vi "load_validation_file.vi"(6 "LUA Validation File":path, 10 "Parameters Tree":refnum<vi>) -> (2 "Vali File Loaded":bool, 3 "# Lines":i32)   [LabVIEW 2019]
uses:
  lib/libSpecValiReader.so
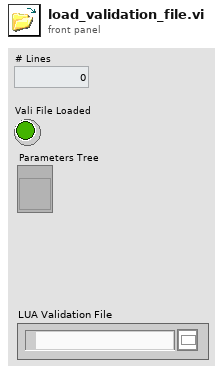
[diagram p1: front panel]
types:
  T1 = cluster{string, string[], "Child Tag":string, i32, "Child Only?":bool, i32}
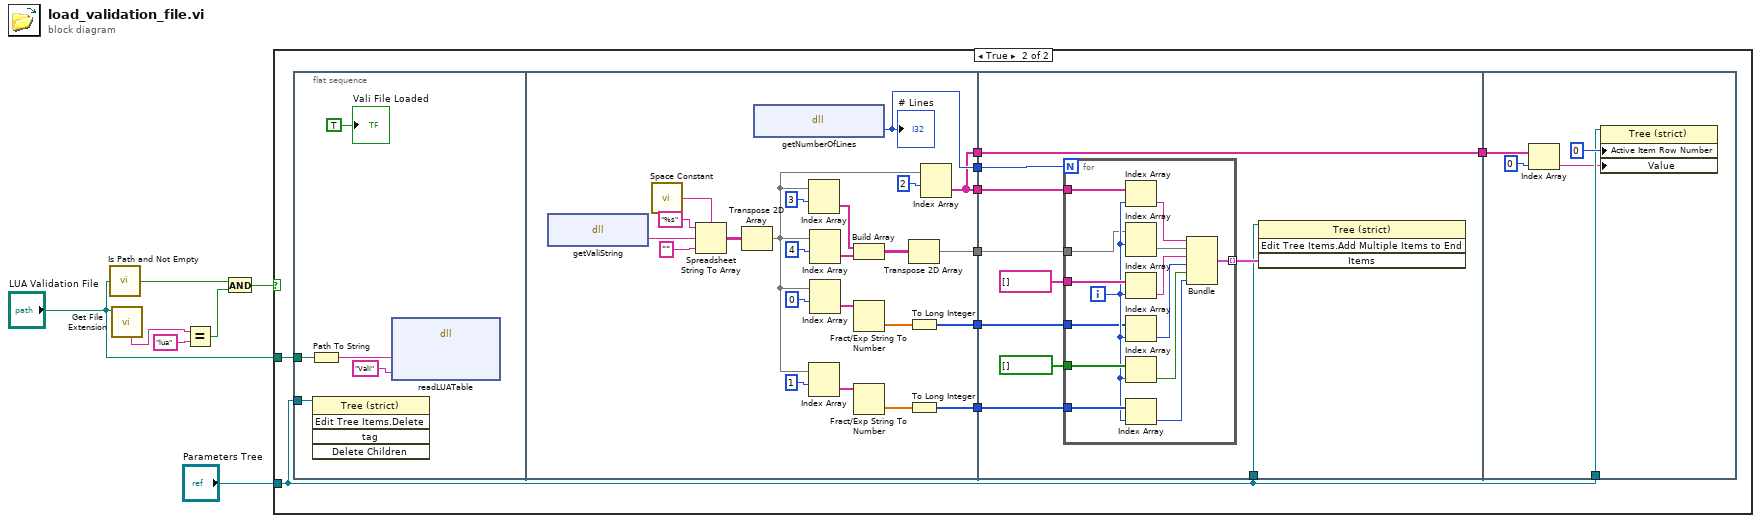
[diagram p0: block diagram]
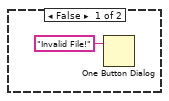
[diagram p2: hidden frame]
diagram:
  n1 = call <vilib>:"Is Path and Not Empty.vi"("path"="LUA Validation File") -> ("Is Path and Not Empty?"=w3:bool)  [unwired: 4 in]
  n2 = call <vilib>:"Get File Extension.vi"("file"="LUA Validation File") -> ("unmodified file extension"=w6:string)  [unwired: 6 in, 4 out]
  n3 = Equal?(x=w6, y="lua") -> (x = y?=w2:bool)
  n4 = And(x=w3, y=w2) -> (x .and. y?=w1:bool)
  n5 = case shown="True" w1 {
    tunnel: "Parameters Tree" -> [_ w10]
    tunnel: "LUA Validation File" -> [_ w9]
    frame False {
      n6 = One Button Dialog(message="Invalid File!") -> ()  [unwired: 1 in, 1 out]
    }
    frame True {
      n7 = flat-sequence {
        tunnel: w10 -> [w20]
        tunnel: w9 -> [w18]
        tunnel: [w41] -> w17
        tunnel: [w36] -> w16
        tunnel: [w32] -> w15
        tunnel: [w25] -> w14
        tunnel: [w25] -> w13
        tunnel: [w23] -> w12
        tunnel: w17 -> [w52]
        tunnel: w10 -> [w51]
        tunnel: w16 -> [w50]
        tunnel: w15 -> [w49]
        tunnel: w14 -> [w48]
        tunnel: [w47] -> w11
        tunnel: w13 -> [w47]
        tunnel: w12 -> [w46]
        tunnel: w10 -> [w72]
        tunnel: w11 -> [w71]
        frame #0 {
          n8 = Path To String(path=w18) -> (string=w19:string)
          n9 = invoke on="Invoke Node" class="Tree (strict)" method="Edit Tree Items.Delete"(reference=w20) -> ()  [unwired: 4 in, 5 out]
          n10 = dll-call lib="home/paul/Schreibtisch/Biogas_plant_setup/lib/libSpecValiReader.so" fn="readLUATable"("filename"=w19, "vali_or_spec"="Vali" ("spec_filename")) -> ()  [unwired: 6 in, 2 out]
          "Vali File Loaded" <- TRUE ("Vali File Loaded")
        }
        frame #1 {
          n11 = dll-call lib="home/paul/Schreibtisch/Biogas_plant_setup/lib/libSpecValiReader.so" fn="getValiString"() -> ("return type"=w45:string)  [unwired: 3 in, 2 out]
          n12 = call <vilib>:"Space Constant.vi"() -> ("String"=w40:string)
          n13 = Spreadsheet String To Array(delimiter (Tab)=w40, format string="%s", spreadsheet string=w45, array type (2D Dbl)="") -> (array=w42:string[][])
          n14 = Transpose 2D Array(2D array=w42) -> (transposed array=w29:string[][])
          n15 = dll-call lib="home/paul/Schreibtisch/Biogas_plant_setup/lib/libSpecValiReader.so" fn="getNumberOfLines"() -> ("numLines"=w41:i32)  [unwired: 3 in, 2 out]
          "# Lines" <- w41
          n16 = Index Array(array=w29, index (row)=3) -> (element=w27:string[])  [unwired: 1 in]
          n17 = Index Array(array=w29, index (row)=1) -> (element=w34:string[])  [unwired: 1 in]
          n18 = Index Array(array=w29, index (row)=4) -> (element=w26:string[])  [unwired: 1 in]
          n19 = Index Array(array=w29, index (row)=0) -> (element=w38:string[])  [unwired: 1 in]
          n20 = Build Array(w27, w26) -> (w24:string[][])
          n21 = Fract/Exp String To Number(string=w38) -> (number=w37:dbl[])  [unwired: 3 in, 1 out]
          n22 = Fract/Exp String To Number(string=w34) -> (number=w33:dbl[])  [unwired: 3 in, 1 out]
          n23 = Transpose 2D Array(2D array=w24) -> (transposed array=w23:string[][])
          n24 = To Long Integer(number=w37) -> (32bit integer=w36:i32[])
          n25 = To Long Integer(number=w33) -> (32bit integer=w32:i32[])
          n26 = Index Array(array=w29, index (row)=2) -> (element=w25:string[])  [unwired: 1 in]
        }
        frame #2 {
          n27 = for {
            N: w52 -> [_]
            tunnel: w48 -> [w69]
            tunnel: string[] [] ("Child Tag") -> [w68]
            tunnel: w50 -> [w56]
            tunnel: bool[] [] ("Child Only?") -> [w67]
            tunnel: w49 -> [w66]
            tunnel: [w60] -> w55 mode=indexing
            tunnel: w46 -> [w58]
            i -> [w59]
            n28 = Index Array(array=w69, index=w59) -> (element=w65:string)
            n29 = Index Array(array=w58, index (row)=w59) -> (element=w57:string[])  [unwired: 1 in]
            n30 = Index Array(array=w68, index=w59) -> (element=w64:string)
            n31 = Index Array(array=w56, index=w59) -> (element=w63:i32)
            n32 = Index Array(array=w67, index=w59) -> (element=w62:bool)
            n33 = Index Array(array=w66, index=w59) -> (element=w61:i32)
            n34 = Bundle(w65, w57, "Child Tag"=w64, w63, "Child Only?"=w62, w61) -> (w60:T1)  [unwired: 1 in]
          }
          n35 = invoke on="Invoke Node" class="Tree (strict)" method="Edit Tree Items.Add Multiple Items to End"(reference=w51, "Items"=w55) -> ()  [unwired: 2 in, 4 out]
        }
        frame #3 {
          n36 = Index Array(array=w71, index=0) -> (element=w70:string)
          n37 = property on="Property Node" class="Tree (strict)"(reference=w72, "Active Item Row Number"=0 ("Active Item:Row Number"), "Value"=w70) -> ()  [unwired: 1 in, 2 out]
        }
      }
    }
  }
